vi "取水点无水样数据存储.vi"(8 "error in (no error)":errorcluster, 9 "数据标识":string, 10 "数据类型":string, 11 "table":string) -> (0 "error out":errorcluster)   [LabVIEW 2016, in "PLC.lvlib"]
uses:
  PLC.lvlib
  <vilib>/Utility/sysdir.llb/System Directory Type.ctl
  <vilib>/addons/database/Connection.llb/DB Tools Open Connec (String).vi
  <vilib>/addons/database/NI_Database_API.lvlib
panel:
  in  "存储变量":T1={"时间标识"=timestamp(0 s since 1904-01-01), "测量模式"="", "数据类型"="N", "水样浓度值"=0.0, "数据标识"="Z"}
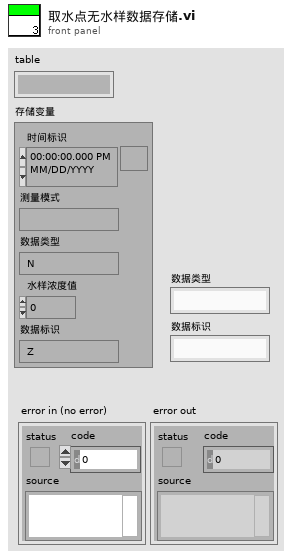
[diagram p1: front panel]
types:
  T1 = cluster{"时间标识":timestamp, "测量模式":string, "数据类型":string, "水样浓度值":dbl, "数据标识":string}
  T2 = typedef "System Directory Type.ctl" = i32
  T3 = typedef "NI_Database_API.lvlib/Conn ObjectReference.ctl" = refnum<k1>
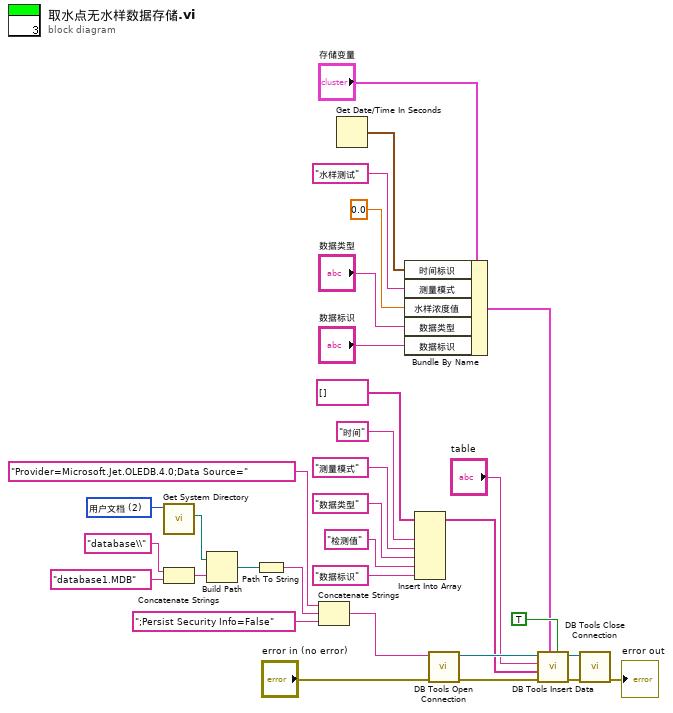
[diagram p0: block diagram]
diagram:
  w29 = T2 2 items=["用户目录"=0, "用户桌面"=1, "用户文档"=2, "用户应用程序数据"=3, "用户设置"=4, "用户临时目录"=5, "公共文档"=6, "公共应用程序数据"=7, "公共设置"=8, "公共缓存"=13, "系统核心库"=9, "系统安装库"=10, "应用程序文件"=11, "启动盘根目录"=12] ("system directory type")
  n1 = call <vilib>:"Get System Directory.vi"("system directory type"=w29) -> ("system directory"=w27:path)  [unwired: 10 in]
  n2 = Concatenate Strings("database\\" ("condition"), "database1.MDB" ("condition")) -> (w21:string)
  n3 = Build Path(base path=w27, name or relative path=w21) -> (appended path=w26:path)
  n4 = Path To String(path=w26) -> (string=w25:string)
  n5 = Concatenate Strings("Provider=Microsoft.Jet.OLEDB.4.0;Data Source=" ("condition"), w25, ";Persist Security Info=False" ("condition")) -> (w23:string)
  n6 = Get Date/Time In Seconds() -> (seconds since 1Jan1904=w4:timestamp)
  n7 = Bundle By Name(cluster="存储变量", "时间标识"=w4, "测量模式"="水样测试", "水样浓度值"=0.0, "数据类型"="数据类型", "数据标识"="数据标识") -> (w6:T1)
  n8 = Insert Into Array(array=string[] [] ("columns"), new element #1="时间" ("新元素/子数组"), new element #2="测量模式" ("新元素/子数组"), new element #3="数据类型" ("新元素/子数组"), new element #4="检测值" ("新元素/子数组"), new element #5="数据标识" ("新元素/子数组")) -> (w13:string[])  [unwired: 1 in]
  n9 = call-poly <vilib>:"DB Tools Open Connection.vi"("error in (no error)"="error in (no error)", "connection information"=w23) -> ("error out"=w19:errorcluster, "connection reference"=w20:T3)  [unwired: 6 in]
  n10 = call <vilib>:"DB Tools Insert Data.vi"("create table? (F)"=TRUE, "data"=w6, "error in (no error)"=w19, "columns"=w13, "table"="table", "connection reference"=w20) -> ("error out"=w31:errorcluster, "connection reference out"=w32:T3)  [unwired: 4 in]
  n11 = call <vilib>:"DB Tools Close Connection.vi"("error in (no error)"=w31, "connection reference"=w32) -> ("error out"=→"error out":errorcluster)  [unwired: 5 in]
